vi "Get Count.vi"(8 "error in (no error)":errorcluster caption="错误输入（无错误）", 11 "雇员名录管理 输入":refnum<class "雇员名录管理.lvclass"> caption="DNL_LabVIEW Object in") -> (0 "error out":errorcluster caption="错误输出", 1 "Count":i32, 3 "雇员名录管理 输出":refnum<class "雇员名录管理.lvclass"> caption="DNL_LabVIEW Object out")   [LabVIEW 2011, in "迭代器.lvlib" / "雇员名录管理.lvclass"]
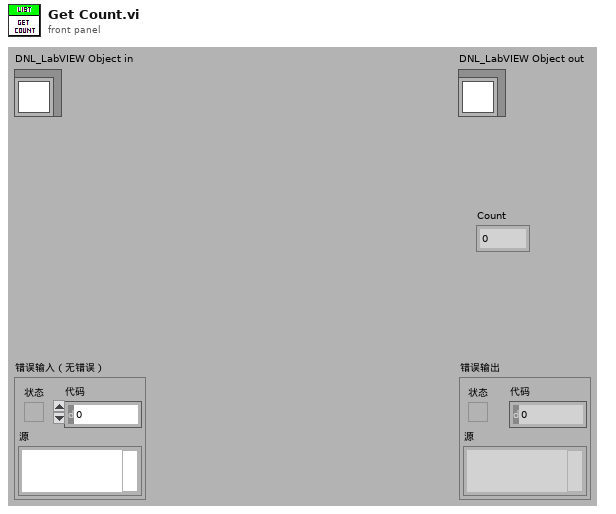
[diagram p1: front panel]
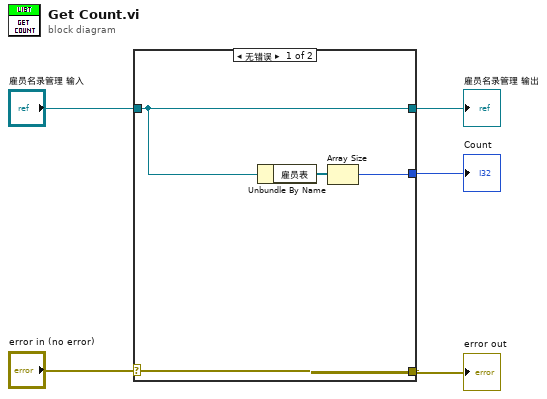
[diagram p0: block diagram]
diagram:
  n1 = case shown="无错误" "error in (no error)" {
    selector: "error in (no error)" -> [w9 w11]
    tunnel: [w9 w11] -> w4
    tunnel: [w8 w10] -> w2
    tunnel: "雇员名录管理 输入" -> [w8 w10]
    tunnel: [w6 _] -> w1
    frame No Error {
      n2 = Unbundle By Name(w8) -> ("雇员表"=w7:refnum<class "雇员.lvclass">[])
      n3 = Array Size(array=w7) -> (size(s)=w6:i32)
    }
    frame Error {
    }
  }
  "error out" <- w4
  "雇员名录管理 输出" <- w2
  "Count" <- w1
